vi "Turret Structure.vi"(0 "AIDeviceRef":T1, 1 "Raw Turret":dbl, 2 "upper limit":dbl=4.5, 3 "lower limit":dbl=0.85, 5 "Turret Case":i32, 7 "Home Speed":dbl=1.0, 9 "Home postion":dbl, 11 "error in (no error)":errorcluster) -> (6 "Turret Output":dbl, 15 "Turret Case Output":dbl)   [LabVIEW 2011]
uses:
  <vilib>/Rock Robotics/WPI/AnalogChannel/WPI_AnalogChannelDevRef.ctl
  <vilib>/Rock Robotics/SystemInterfaces/Typedef/FPGA_TypedefAnalogModule.ctl
  <vilib>/Rock Robotics/SystemInterfaces/AI/FPGA_AIChannel.ctl
  <vilib>/addons/control/pid/pid.llb/PID (DBL).vi
  <vilib>/addons/control/pid/NI_PID_pid.lvlib
panel:
  in  "-1/1 per degree":dbl=0.05
  in  "Volts per degree":dbl=0.0166666666666667
  in  "PID Gains":T4={"proportional gain (Kc)"=1.0, "integral time (Ti, min)"=0.01, "derivative time (Td, min)"=0.0} {"derivative time (Td, min)" format="%.3f"; "integral time (Ti, min)" format="%.3f"; "proportional gain (Kc)" format="%.3f"}
  out "Waveform Chart":dynamicdata(graph)
  in  "PID Enable":bool
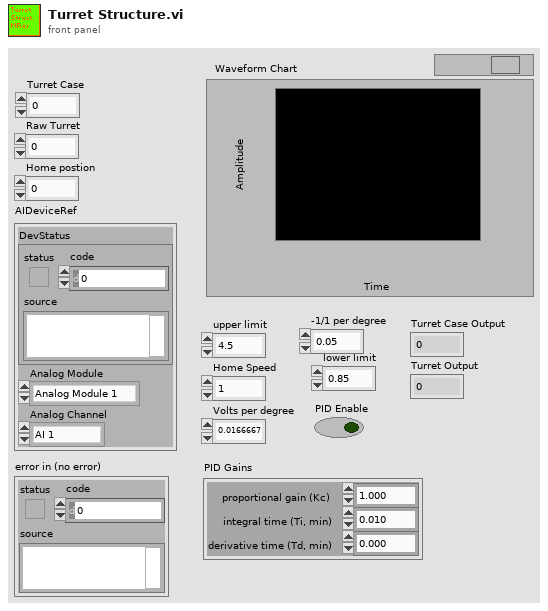
[diagram p1: front panel]
types:
  T1 = typedef "WPI_AnalogChannelDevRef.ctl" = cluster{"DevStatus":errorcluster, "Analog Module":T2, "Analog Channel":T3}
  T2 = typedef "FPGA_TypedefAnalogModule.ctl" = enum16{"Analog Module 1", "Analog Module 2"}
  T3 = typedef "FPGA_AIChannel.ctl" = enum8{"AI 1", "AI 2", "AI 3", "AI 4", "AI 5", "AI 6", "AI 7", "AI 8", "Invalid"}
  T4 = cluster{"proportional gain (Kc)":dbl, "integral time (Ti, min)":dbl, "derivative time (Td, min)":dbl}
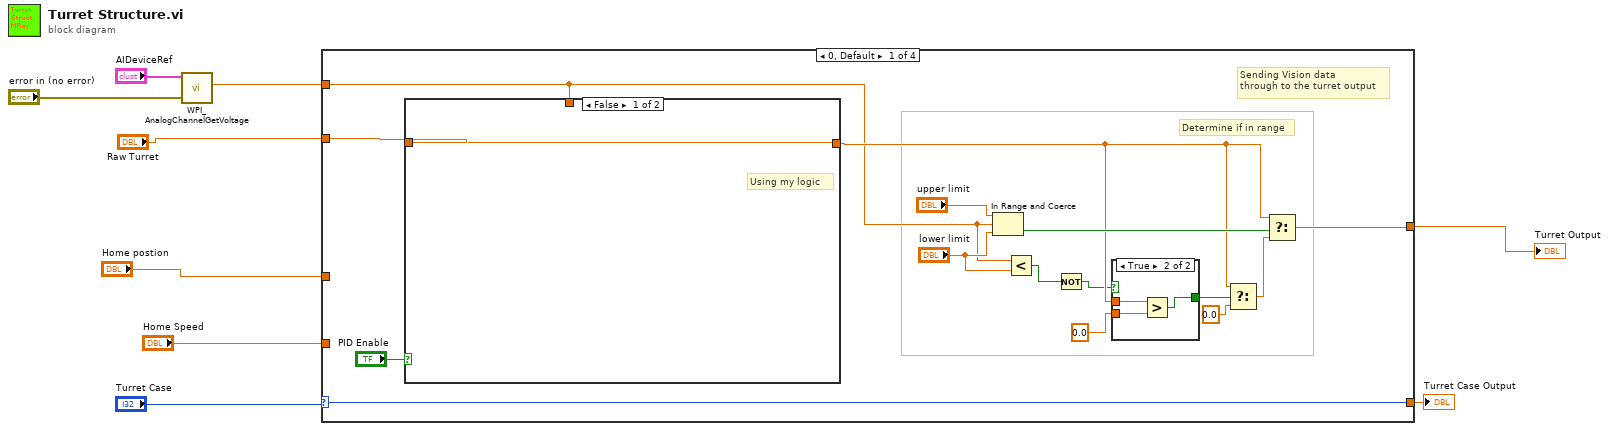
[diagram p0: block diagram]
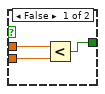
[diagram p2: hidden frame]
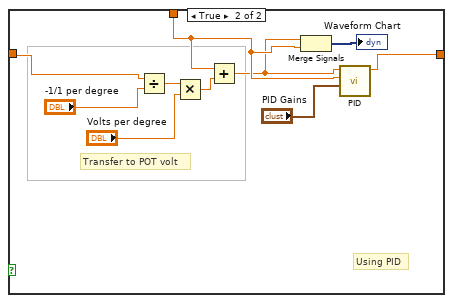
[diagram p3: hidden frame]
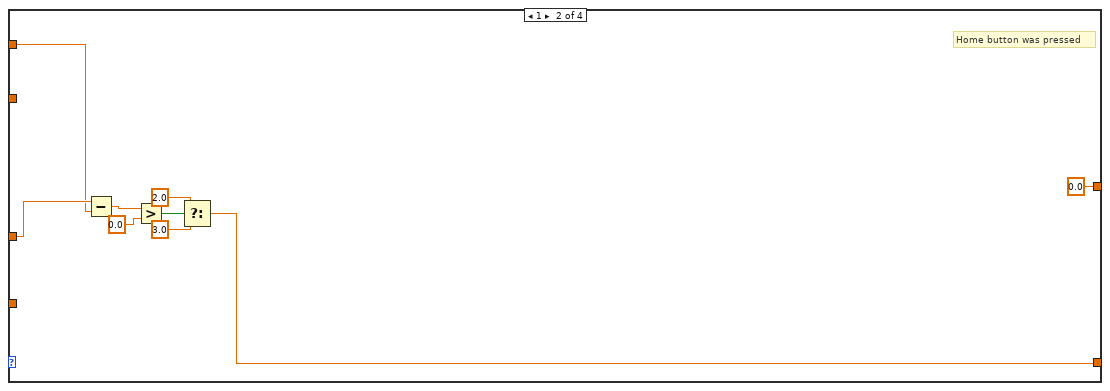
[diagram p4: hidden frame]
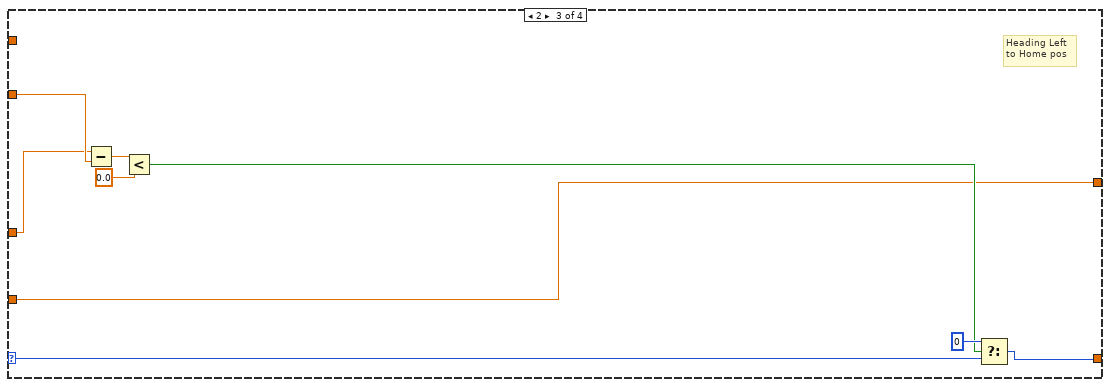
[diagram p5: hidden frame]
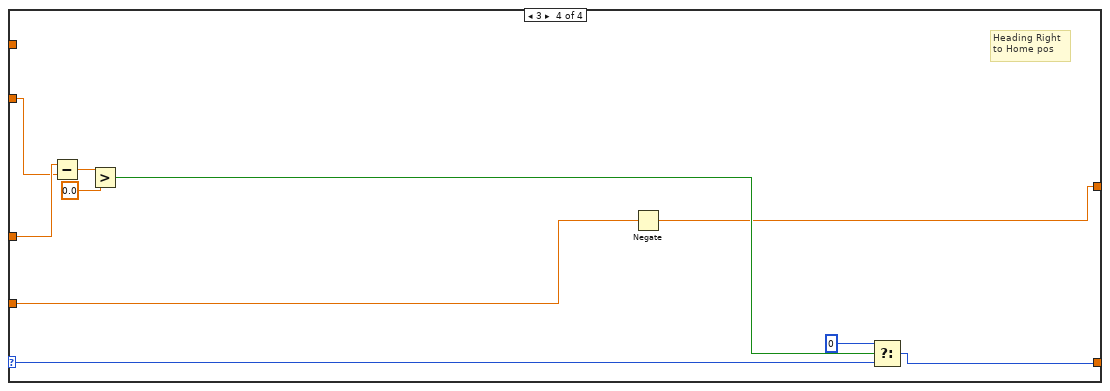
[diagram p6: hidden frame]
diagram:
  n1 = call <vilib>:"WPI_AnalogChannelGetVoltage.vi"("error in (no error)"="error in (no error)", "AIDeviceRef"="AIDeviceRef") -> ("Voltage"=w9:dbl)  [unwired: 7 in, 2 out]
  n2 = case shown="0, Default" "Turret Case" {
    selector: "Turret Case" -> [w13 _ w54 w64]
    tunnel: w9 -> [w12 w44 _ _]
    tunnel: "Raw Turret" -> [w21 _ w57 w66]
    tunnel: [w14 0.0 ("Home Speed 2") w51 w60] -> w8
    tunnel: "Home postion" -> [_ w45 w56 w67]
    tunnel: [w13 w43 w53 w63] -> w1
    tunnel: "Home Speed" -> [_ _ w51 w61]
    frame 0, Default {
      # "Determine if in range"
      # "Sending Vision data\nthrough to the turret output"
      n3 = case shown="False" "PID Enable" {
        tunnel: w21 -> [w31 w40]
        tunnel: [w31 w35] -> w17
        tunnel: w12 -> [_ w33]
        frame False {
          # "Using my logic"
        }
        frame True {
          # "Transfer to POT volt"
          # "Using PID"
          n4 = Divide(x=w40, y="-1/1 per degree") -> (x/y=w39:dbl)
          n5 = Multiply(x=w39, y="Volts per degree") -> (x*y=w37:dbl)
          n6 = Add(x=w33, y=w37) -> (x+y=w32:dbl)
          n7 = Merge Signals(w32, w33) -> (→"Waveform Chart":dynamicdata)
          n8 = call-poly <vilib>:"PID.vi"("PID gains"="PID Gains", "process variable"=w33, "setpoint"=w32) -> ("output"=w35:dbl)  [unwired: 7 in, 1 out]
        }
      }
      n9 = In Range and Coerce(upper limit="upper limit", x=w12, lower limit="lower limit") -> (In Range?=w22:bool)  [unwired: 1 out]
      n10 = Less?(x=w12, y="lower limit") -> (x < y?=w11:bool)
      n11 = Not(x=w11) -> (.not. x?=w10:bool)
      n12 = case shown="True" w10 {
        tunnel: 0.0 -> [w26 w30]
        tunnel: [w25 w29] -> w18
        tunnel: w17 -> [w27 w28]
        frame False {
          n13 = Less?(x=w27, y=w26) -> (x < y?=w25:bool)
        }
        frame True {
          n14 = Greater?(x=w28, y=w30) -> (0:w29:bool)
        }
      }
      n15 = Select(t=w17, s=w18, f=0.0) -> (s? t:f=w16:dbl)
      n16 = Select(t=w17, s=w22, f=w16) -> (s? t:f=w14:dbl)
    }
    frame 1 {
      # "Home button was pressed"
      n17 = Subtract(x=w45, y=w44) -> (x-y=w46:dbl)
      n18 = Greater?(x=w46, y=0.0) -> (0:w48:bool)
      n19 = Select(t=2.0, s=w48, f=3.0) -> (s? t:f=w43:dbl)
    }
    frame 2 {
      # "Heading Left\nto Home pos"
      n20 = Subtract(x=w56, y=w57) -> (x-y=w58:dbl)
      n21 = Less?(x=w58, y=0.0) -> (x < y?=w52:bool)
      n22 = Select(t=0, s=w52, f=w54) -> (s? t:f=w53:i32)
    }
    frame 3 {
      # "Heading Right\nto Home pos"
      n23 = Subtract(x=w67, y=w66) -> (x-y=w68:dbl)
      n24 = Greater?(x=w68, y=0.0) -> (0:w62:bool)
      n25 = Negate(x=w61) -> (-x=w60:dbl)
      n26 = Select(t=0, s=w62, f=w64) -> (s? t:f=w63:i32)
    }
  }
  "Turret Case Output" <- w1
  "Turret Output" <- w8
